vi "Project_Get Named Build Specification.vi"(7 "Close project reference(T)":bool=TRUE, 8 "error in(no error)":errorcluster, 9 "Target Name(\"\"> My Computer)":string, 10 "Build Specification Name":string, 11 "Project Path":path) -> (0 "error out":errorcluster, 1 "Success?":bool, 2 "Build Spec reference":refnum<vi>, 3 "Project reference (if not closed)":refnum<vi>)   [LabVIEW 2019, in "ProjectBuilder.lvlib"]
doc: "Get a build specification reference for a named specification on the specified target."
uses:
  ProjectBuilder.lvlib
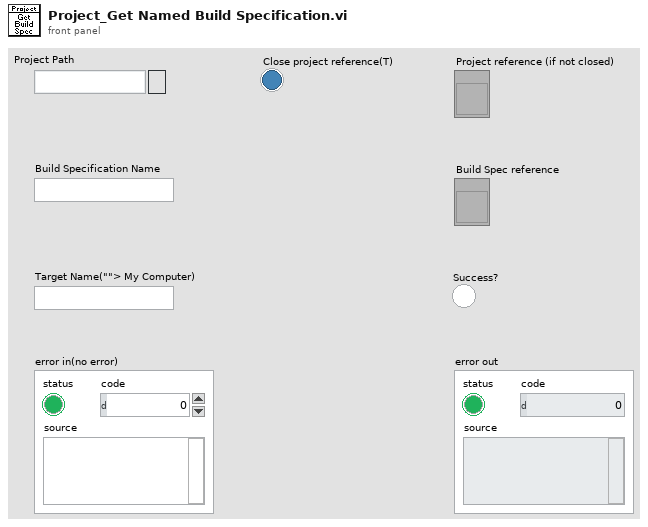
[diagram p1: front panel]
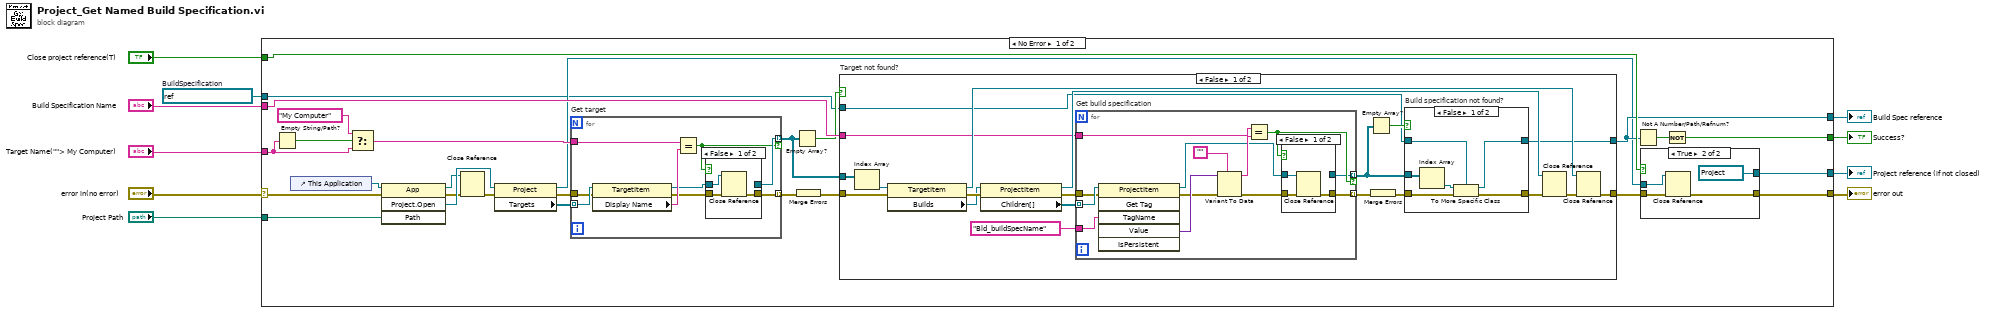
[diagram p0: block diagram]
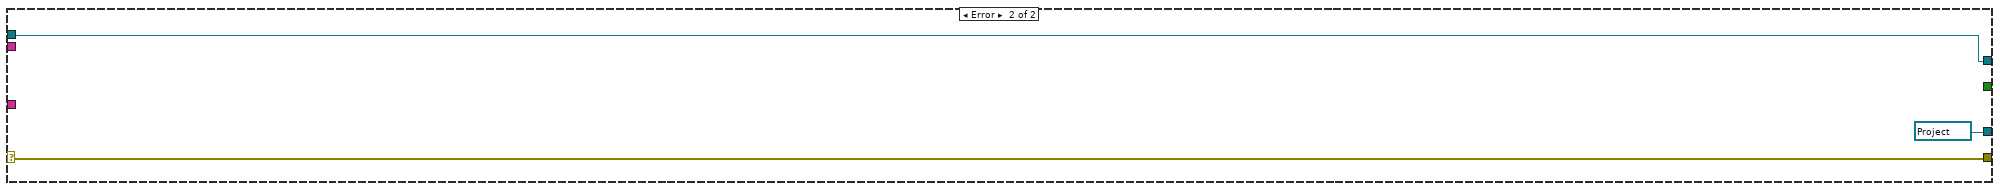
[diagram p7: hidden frame]
diagram:
  w1 = refnum<vi> refnum  # BuildSpecification
  n1 = case shown="No Error" "error in(no error)" {
    selector: "error in(no error)" -> [w36 w108]
    tunnel: "Project Path" -> [w37 _]
    tunnel: "Target Name(\"\"> My Computer)" -> [w35 _]
    tunnel: "Build Specification Name" -> [w34 _]
    tunnel: "Close project reference(T)" -> [w18 _]
    tunnel: [w17 w108] -> w5
    tunnel: [w16 w106] -> w4
    tunnel: [w14 _] -> w3
    tunnel: [w12 refnum<vi> refnum ("Project:Open")] -> w2
    tunnel: w1 -> [w11 w106]
    frame No Error {
      n2 = Empty String/Path?(string/path=w35) -> (empty?=w28:bool)
      n3 = control-ref of="This Application"() -> (w24:refnum<vi>)
      n4 = Select(t="My Computer", s=w28, f=w35) -> (s? t:f=w29:string)
      n5 = invoke class="App" method="Project.Open"(reference=w24, error in=w36, "Path"=w37) -> (reference out=w21:refnum<vi>, error out=w20:errorcluster, "Project:Open"=w26:refnum<vi>)  [unwired: 1 in, 1 out]
      n6 = Close Reference(reference=w21, error in (no error)=w20) -> (error out=w19:errorcluster)
      n7 = property class="Project"(reference=w26, error in=w19) -> (reference out=w13:refnum<vi>, error out=w32:errorcluster, "Targets"=w30:refnum<vi>[])
      n8 = for "Get target" {
        tunnel: w30 -> [w100] mode=indexing
        tunnel: w29 -> [w98]
        tunnel: [w96] -> w23 mode=indexing if=w92
        tunnel: w32 -> [w95]
        tunnel: [w93] -> w31 mode=indexing
        n9 = property class="TargetItem"(reference=w100, error in=w95) -> (reference out=w97:refnum<vi>, error out=w94:errorcluster, "Display Name"=w99:string)
        n10 = Equal?(x=w98, y=w99) -> (x = y?=w92:bool)
        n11 = case shown="False" w92 {
          tunnel: [_ w105] -> w96
          tunnel: w97 -> [w103 w105]
          tunnel: w94 -> [w102 w104]
          tunnel: [w101 w104] -> w93
          frame False {
            n12 = Close Reference(reference=w103, error in (no error)=w102) -> (error out=w101:errorcluster)
          }
          frame True {
          }
        }
      }
      n13 = Empty Array?(array=w23) -> (empty?=w22:bool)
      n14 = Merge Errors(w31) -> (w33:errorcluster)
      n15 = case "Target not found?" shown="False" w22 {
        tunnel: w33 -> [w63 w91]
        tunnel: w23 -> [w61 _]
        tunnel: [w55 w91] -> w27
        tunnel: w34 -> [w48 _]
        tunnel: [w45 w90] -> w16
        tunnel: w11 -> [w44 w90]
        frame False {
          n16 = Index Array(array=w61) -> (element=w50:refnum<vi>)  [unwired: 1 in]
          n17 = property class="TargetItem"(reference=w50, error in=w63) -> (reference out=w62:refnum<vi>, error out=w56:errorcluster, "Builds"=w51:refnum<vi>)
          n18 = property class="ProjectItem"(reference=w51, error in=w56) -> (reference out=w54:refnum<vi>, error out=w59:errorcluster, "Children[]"=w57:refnum<vi>[])
          n19 = for "Get build specification" {
            tunnel: w57 -> [w84] mode=indexing
            tunnel: "Bld_buildSpecName" ("String") -> [w83]
            tunnel: w48 -> [w79]
            tunnel: w59 -> [w78]
            tunnel: [w75] -> w47 mode=indexing if=w77
            tunnel: [w72] -> w58 mode=indexing
            n20 = invoke class="ProjectItem" method="Get Tag"(reference=w84, error in=w78, "TagName"=w83) -> (reference out=w76:refnum<vi>, error out=w74:errorcluster, "Value"=w82:variant)  [unwired: 3 in, 3 out]
            n21 = Variant To Data(error in=w74, type="", Variant=w82) -> (data=w80:string, error out=w73:errorcluster)
            n22 = Equal?(x=w79, y=w80) -> (x = y?=w77:bool)
            n23 = case shown="False" w77 {
              tunnel: [_ w89] -> w75
              tunnel: w76 -> [w87 w89]
              tunnel: w73 -> [w86 w88]
              tunnel: [w85 w88] -> w72
              frame False {
                n24 = Close Reference(reference=w87, error in (no error)=w86) -> (error out=w85:errorcluster)
              }
              frame True {
              }
            }
          }
          n25 = Empty Array?(array=w47) -> (empty?=w46:bool)
          n26 = Merge Errors(w58) -> (w60:errorcluster)
          n27 = case "Build specification not found?" shown="False" w46 {
            tunnel: w60 -> [w69 w71]
            tunnel: w47 -> [w68 _]
            tunnel: [w66 w71] -> w52
            tunnel: [w65 w70] -> w45
            tunnel: w44 -> [w64 w70]
            frame False {
              n28 = Index Array(array=w68) -> (element=w67:refnum<vi>)  [unwired: 1 in]
              n29 = To More Specific Class(target class=w64, reference=w67, error in=w69) -> (specific class reference=w65:refnum<vi>, error out=w66:errorcluster)
            }
            frame True {
            }
          }
          n30 = Close Reference(reference=w54, error in (no error)=w52) -> (error out=w53:errorcluster)
          n31 = Close Reference(reference=w62, error in (no error)=w53) -> (error out=w55:errorcluster)
        }
        frame True {
        }
      }
      n32 = Not A Number/Path/Refnum?(number/path/refnum=w16) -> (NaN/Path/Refnum?=w15:bool)
      n33 = case shown="True" w18 {
        tunnel: w13 -> [w38 w43]
        tunnel: w27 -> [w39 w42]
        tunnel: [w39 w41] -> w17
        tunnel: [w38 refnum<vi> refnum ("Project:Open")] -> w12
        frame False {
        }
        frame True {
          n34 = Close Reference(reference=w43, error in (no error)=w42) -> (error out=w41:errorcluster)
        }
      }
      n35 = Not(x=w15) -> (.not. x?=w14:bool)
    }
    frame Error {
    }
  }
  "Project reference (if not closed)" <- w2
  "error out" <- w5
  "Build Spec reference" <- w4
  "Success?" <- w3
